vi "Actor Core.vi"(8 "error in":errorcluster, 11 "TestQList in":refnum<class "TestQList.lvclass">) -> (0 "error out":errorcluster, 3 "Actor out":refnum<class "Actor.lvclass">)   [LabVIEW 2019, in "TestQList.lvclass"]
doc: "(<B>Filename</B>: Actor Framework.lvlib:Actor.lvclass:Actor Core.vi)\n\nReceives messages to the actor, reacts to them, and initiates any error handling that may shut the actor down.\n\nDescendant classes may override this VI to append parallel tasks for the actor to complete while it handles messages. Overrides use the Call Parent Method node."
uses:
  TestQList.lvclass
  C:/Program Files/National Instruments/LabVIEW 2019/vi.lib/ActorFramework/Actor/Actor.lvclass
  <vilib>/ActorFramework/Actor/Actor.lvclass
  Queued Listbox.xctl
  <vilib>/ActorFramework/Actor/Actor.lvclass/Actor.ctl
  <vilib>/ActorFramework/Message Enqueuer/Message Enqueuer.lvclass/Message Enqueuer.ctl
  <vilib>/ActorFramework/Message Enqueuer/Init from Existing Queue.vi
  <vilib>/ActorFramework/Message Enqueuer/Enqueue.vi
  <vilib>/ActorFramework/Stop Msg/Stop Msg.lvclass
  C:/Program Files/National Instruments/LabVIEW 2019/vi.lib/ActorFramework/Message/Message.lvclass
  <vilib>/ActorFramework/Message Priority Queue/Priority Enqueue.vi
  <vilib>/ActorFramework/Message Enqueuer/Message Enqueuer.lvclass
panel:
  in  "Stop Button":bool
  in  "Queued Listbox":string[](xcontrol)
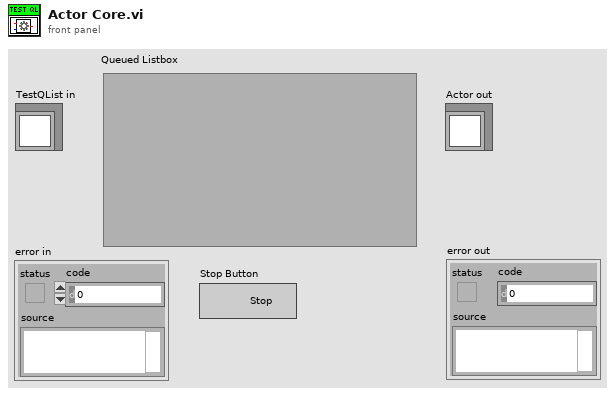
[diagram p1: front panel]
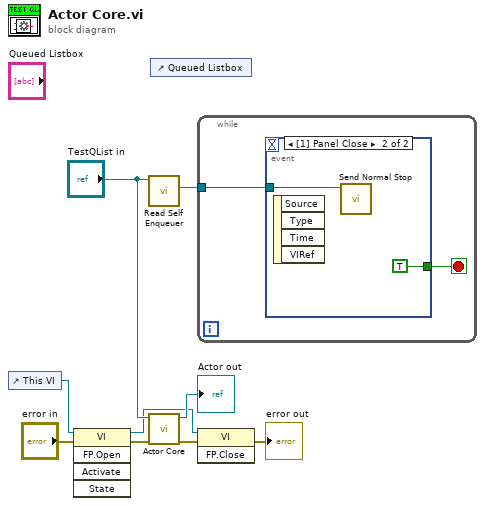
[diagram p0: block diagram]
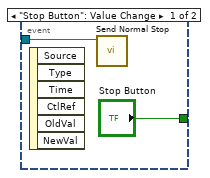
[diagram p2: hidden frame]
diagram:
  n1 = control-ref of="This VI"() -> (w6:refnum<vi>)
  n2 = invoke class="VI" method="FP.Open"(reference=w6, error in="error in") -> (reference out=w2:refnum<vi>, error out=w4:errorcluster)  [unwired: 3 in, 3 out]
  n3 = call <vilib>:"Read Self Enqueuer.vi"("Actor"="TestQList in") -> ("Self Enqueuer"=w7:refnum<class "Message Enqueuer.lvclass">)  [unwired: 10 in]
  n4 = call-parent "Actor Core.vi"("error in"=w4, "Actor in"="TestQList in") -> ("error out"=w3:errorcluster, "Actor out"=→"Actor out":refnum<class "Actor.lvclass">)  [unwired: 8 in]
  n5 = control-ref of="Queued Listbox"() -> ()  [unwired: 1 out]
  n6 = while {
    tunnel: w7 -> [w11]
    stop <- w10 stop-if-true
    n7 = event shown="[1] Panel Close" {
      selector: _ -> [_ _]
      dyn-events: _ -> [_ _]
      timeout: _ -> [_ _]
      tunnel: w11 -> [w13 w15]
      tunnel: ["Stop Button" TRUE ("Stop Button")] -> w10
      event "Stop Button": Value Change {
        n8 = event-data() -> ()  [unwired: 1 in, 6 out]
        n9 = call <vilib>:"Send Normal Stop.vi"("Message Enqueuer"=w13) -> ()  [unwired: 10 in, 1 out]
      }
      event Panel Close {
        n10 = event-data() -> ()  [unwired: 1 in, 4 out]
        n11 = call <vilib>:"Send Normal Stop.vi"("Message Enqueuer"=w15) -> ()  [unwired: 10 in, 1 out]
      }
    }
  }
  n12 = invoke class="VI" method="FP.Close"(reference=w2, error in=w3) -> (error out=→"error out":errorcluster)  [unwired: 1 in, 2 out]
